vi "Surface_ColorScale.vi"(4 "ColorMapAutoScale":bool=TRUE, 6 "Min":dbl=-0.8, 7 "Max":dbl=0.6, 8 "3D Surface_":refnum<k7>(container)) -> (0 "Color Map out":u32[](array[colorbox])=[0, 16711935, 255, 65535, 65280, 16776960, 16744448, 16711680, 16777215], 2 "Min 2":dbl=-0.8, 3 "Max 2":dbl=0.6, 5 "Color Value":dbl[](array[numeric])=[-0.8, -0.625, -0.45000000000000007, -0.27500000000000013, -0.10000000000000009, 0.07499999999999996, 0.24999999999999978, 0.4249999999999998, 0.5999999999999999])   [LabVIEW 2018]
panel:
  in  "Color Map":u32[](array[colorbox])=[0, 16711935, 255, 65535, 65280, 16776960, 16744448, 16711680, 16777215]
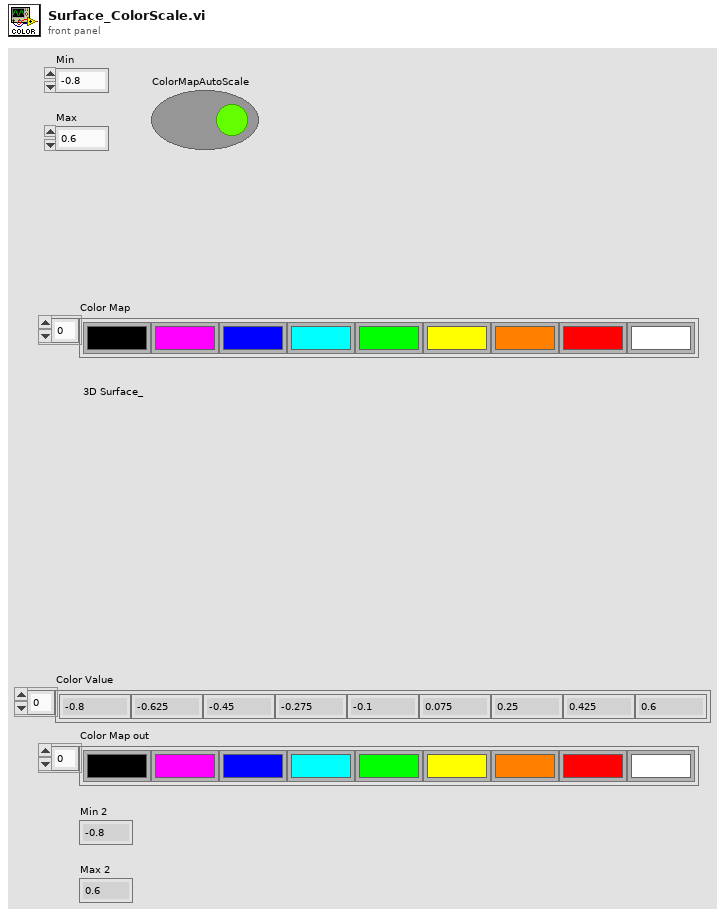
[diagram p1: front panel]
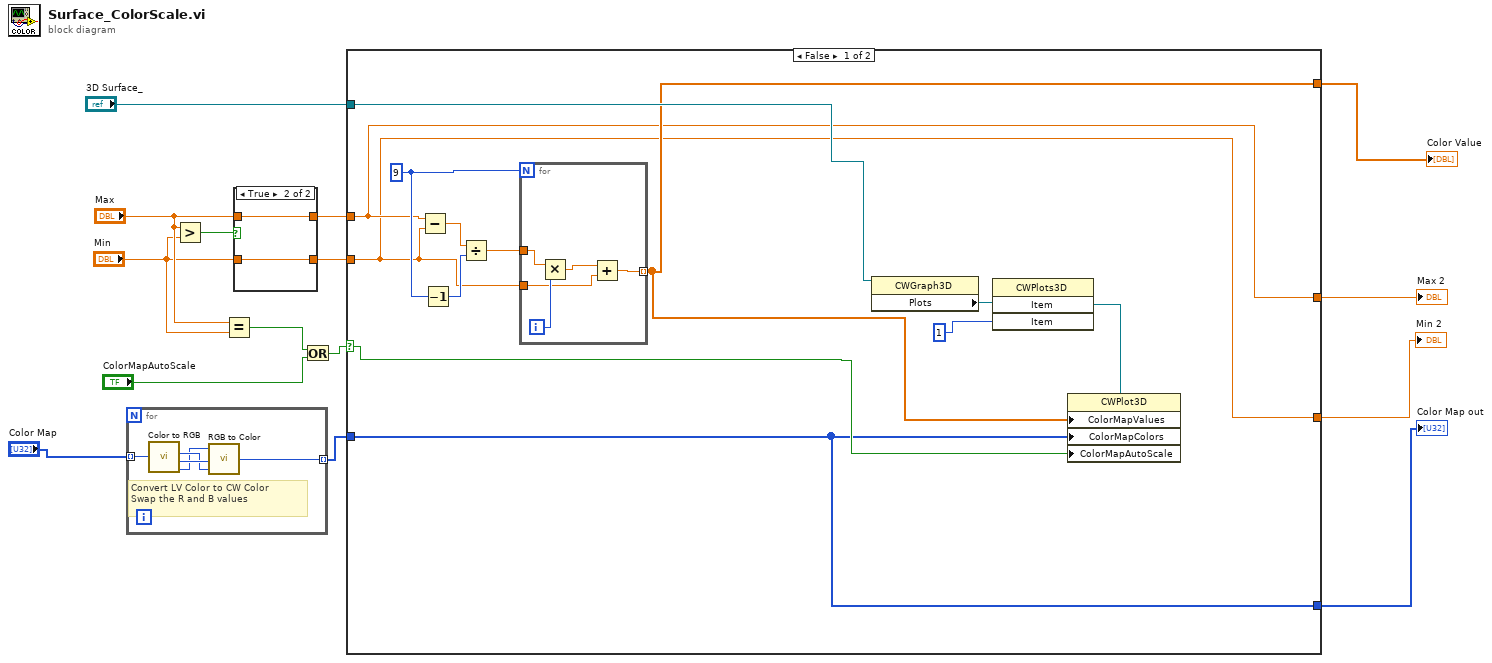
[diagram p0: block diagram]
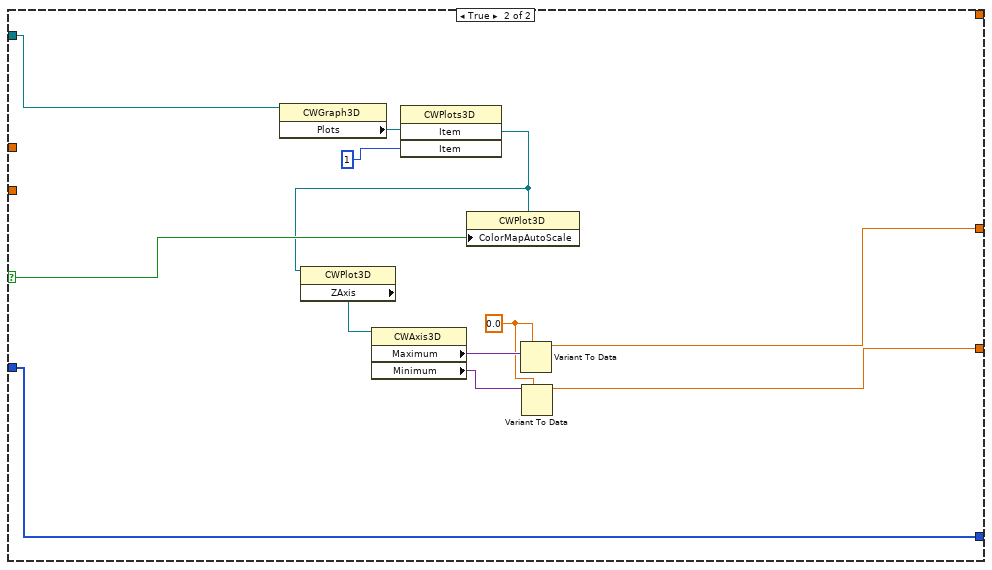
[diagram p3: hidden frame]
diagram:
  n1 = for {
    tunnel: "Color Map" -> [w18] mode=indexing
    tunnel: [w17] -> w10 mode=indexing
    # "Convert LV Color to CW Color\nSwap the R and B values"
    n2 = call <vilib>:"Color to RGB.vi"("Color"=w18) -> ("R"=w19:u8, "G"=w20:u8, "B"=w16:u8)  [unwired: 1 out]
    n3 = call <vilib>:"RGB to Color.vi"("B"=w19, "G"=w20, "R"=w16) -> ("Color"=w17:u32)
  }
  n4 = Greater?(x="Max", y="Min") -> (0:w4:bool)
  n5 = Equal?(x="Max", y="Min") -> (x = y?=w1:bool)
  n6 = case shown="True" w4 {
    tunnel: [w21 w24] -> w6
    tunnel: "Max" -> [w22 w24]
    tunnel: [w22 w23] -> w5
    tunnel: "Min" -> [w21 w23]
    frame False {
    }
    frame True {
    }
  }
  n7 = Or(x=w1, y="ColorMapAutoScale") -> (x .or. y?=w7:bool)
  n8 = case shown="False" w7 {
    selector: w7 -> [w28 w47]
    tunnel: "3D Surface_" -> [w37 w48]
    tunnel: [w32 _] -> w14
    tunnel: w6 -> [w27 _]
    tunnel: w5 -> [w26 _]
    tunnel: [w27 w45] -> w13
    tunnel: [w26 w44] -> w12
    tunnel: w10 -> [w25 w43]
    tunnel: [w25 w43] -> w9
    frame False {
      w36 = 9
      n9 = Subtract(x=w27, y=w26) -> (x-y=w35:dbl)
      n10 = Decrement(x=w36) -> (x-1=w34:i32)
      n11 = Divide(x=w35, y=w34) -> (x/y=w33:dbl)
      n12 = for {
        N: w36 -> [_]
        tunnel: [w42] -> w32 mode=indexing
        tunnel: w33 -> [w41]
        tunnel: w26 -> [w38]
        i -> [w40]
        n13 = Multiply(x=w41, y=w40) -> (x*y=w39:dbl)
        n14 = Add(x=w39, y=w38) -> (x+y=w42:dbl)
      }
      n15 = property class="CWGraph3D"(reference=w37) -> ("Plots"=w30:refnum<k7>)  [unwired: 1 in, 2 out]
      n16 = invoke class="CWPlots3D" method="Item"(reference=w30, "Item"=1) -> ("Item"=w29:refnum<k7>)  [unwired: 2 in, 3 out]
      n17 = property class="CWPlot3D"(reference=w29, "ColorMapValues"=w32, "ColorMapColors"=w25, "ColorMapAutoScale"=w28) -> ()  [unwired: 1 in, 2 out]
    }
    frame True {
      w50 = 0.0
      n18 = property class="CWGraph3D"(reference=w48) -> ("Plots"=w53:refnum<k7>)  [unwired: 1 in, 2 out]
      n19 = invoke class="CWPlots3D" method="Item"(reference=w53, "Item"=1) -> ("Item"=w46:refnum<k7>)  [unwired: 2 in, 3 out]
      n20 = property class="CWPlot3D"(reference=w46) -> ("ZAxis"=w52:refnum<k7>)  [unwired: 1 in, 2 out]
      n21 = property class="CWAxis3D"(reference=w52) -> ("Maximum"=w51:variant, "Minimum"=w49:variant)  [unwired: 1 in, 2 out]
      n22 = property class="CWPlot3D"(reference=w46, "ColorMapAutoScale"=w47) -> ()  [unwired: 1 in, 2 out]
      n23 = Variant To Data(type=w50, Variant=w51) -> (data=w45:dbl)  [unwired: 1 in, 1 out]
      n24 = Variant To Data(type=w50, Variant=w49) -> (data=w44:dbl)  [unwired: 1 in, 1 out]
    }
  }
  "Color Value" <- w14
  "Color Map out" <- w9
  "Min 2" <- w12
  "Max 2" <- w13
